vi "BOC_type-determain.vi"(0 "paramUnicorn_in":T4, 1 "UI_in":T1, 2 "TCP_conn":bool) -> (6 "paramUnicorn_out":T4={"conParam"={"ReadIntParam"=TRUE, "ReadDescrParam"=FALSE, "ReadFloatParam"=TRUE, "debug"=FALSE, "ReadJSON"=TRUE, "IP_address"="192.168.1.216", "N_attempts"=3, "type_con"=enum."TCP", "MB_address"=1, "VISA"="COM1", "connection ID"=refnum, "nameDevices"="", "timeout"=3000, "port"=2000, "type_version"="0F0C0001", "baud_rate"=115200, "VersionControl"=FALSE, "TCP_conn"=FALSE, "WindowSize"=700}, "Param"={"NumParam"={"NTelem"=0, "NInt"=0, "NFloat"=0, "NTable"=0}, "ParamInt"=[], "Telemetry"=[], "Table"=[], "ParamFloat"=[]}}, 7 "UI_out":T1)   [LabVIEW 2017]
uses:
  Unicorn Labview Library/Control/unicorn_Param.ctl
  Unicorn Labview Library/Control/unicorn_conn.ctl
  Unicorn Labview Library/Control/unicorn_JSON.ctl
  Unicorn Labview Library/Control/unicorn_ParamInt.ctl
  Unicorn Labview Library/Control/unicorn_Telemetry.ctl
  Unicorn Labview Library/Control/unicorn_Table.ctl
  Unicorn Labview Library/Control/unicorn_ParamFloat.ctl
  ui.ctl
  classes/dc_power_supply/DC_power_supply.lvclass
  classes/report/Report.lvclass
  ui_buttons.ctl
  types/boc_type.ctl
  <vilib>/regexp/Match Regular Expression.xnode
  Unicorn Labview Library/Unicorn Library.lvlib
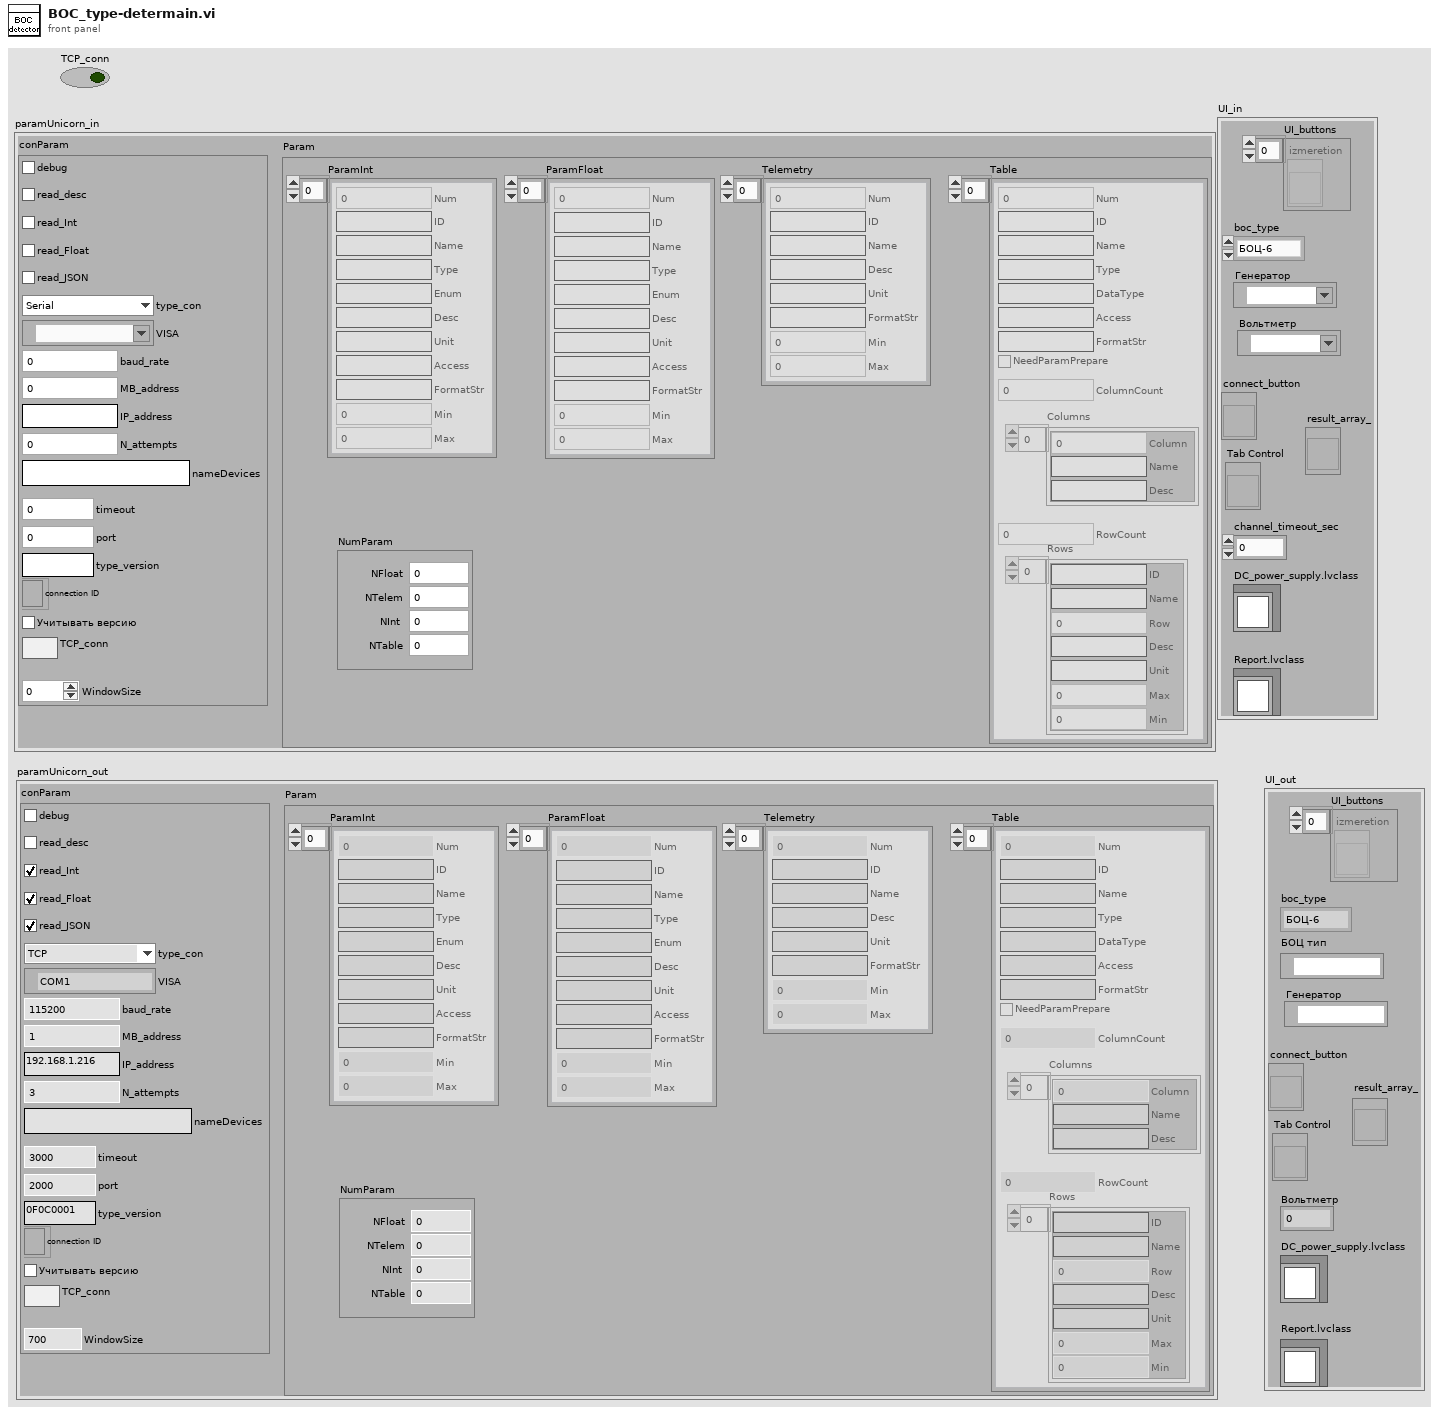
[diagram p1: front panel]
types:
  T1 = typedef "ui.ctl" = cluster{"UI_buttons":T2, "Tab Control":refnum<vi>, "connect_button":refnum<vi>, "generator":refnum<visa-resource-name>, "voltmetr":refnum<visa-resource-name>, "channel_timeout_sec":dbl, "boc_type":T3, "result_array_":refnum<vi>, "DC_power_supply.lvclass":refnum<class "DC_power_supply.lvclass">, "Report.lvclass":refnum<class "Report.lvclass">}
  T2 = typedef "ui_buttons.ctl" = refnum<vi>[]
  T3 = typedef "boc_type.ctl" = enum16{"БОЦ-6", "БОЦ-12"}
  T4 = typedef "Unicorn Library.lvlib/unicorn_Param.ctl" = cluster{"conParam":T5, "Param":T6}
  T5 = typedef "Unicorn Library.lvlib/unicorn_conn.ctl" = cluster{"ReadIntParam":bool, "ReadDescrParam":bool, "ReadFloatParam":bool, "debug":bool, "ReadJSON":bool, "IP_address":string, "N_attempts":i32, "type_con":enum16{"Serial", "TCP"}, "MB_address":i32, "VISA":refnum<visa-resource-name>, "connection ID":refnum<k5>, "nameDevices":string, "timeout":i32, "port":u16, "type_version":string, "baud_rate":u32, "VersionControl":bool, "TCP_conn":bool, "WindowSize":i32}
  T6 = typedef "Unicorn Library.lvlib/unicorn_JSON.ctl" = cluster{"NumParam":cluster{"NTelem":i32, "NInt":i32, "NFloat":i32, "NTable":i32}, "ParamInt":T7, "Telemetry":T8, "Table":T9, "ParamFloat":T10}
  T7 = typedef "Unicorn Library.lvlib/unicorn_ParamInt.ctl" = cluster{"ID":string, "Num":i32, "Name":string, "Type":string, "Enum":string, "Desc":string, "Unit":string, "Access":string, "FormatStr":string, "Min":i32, "Max":i32}[]
  T8 = typedef "Unicorn Library.lvlib/unicorn_Telemetry.ctl" = cluster{"ID":string, "Num":i32, "Name":string, "Desc":string, "Unit":string, "FormatStr":string, "Min":i32, "Max":i32}[]
  T9 = typedef "Unicorn Library.lvlib/unicorn_Table.ctl" = cluster{"Num":i32, "Access":string, "ColumnCount":i32, "NeedParamPrepare":bool, "Columns":cluster{"Column":i32, "Desc":string, "Name":string}[], "DataType":string, "FormatStr":string, "ID":string, "Name":string, "RowCount":i32, "Rows":cluster{"Desc":string, "ID":string, "Max":i32, "Min":i32, "Name":string, "Row":i32, "Unit":string}[], "Type":string}[]
  T10 = typedef "Unicorn Library.lvlib/unicorn_ParamFloat.ctl" = cluster{"ID":string, "Num":i32, "Name":string, "Type":string, "Enum":string, "Desc":string, "Unit":string, "Access":string, "FormatStr":string, "Min":i32, "Max":i32}[]
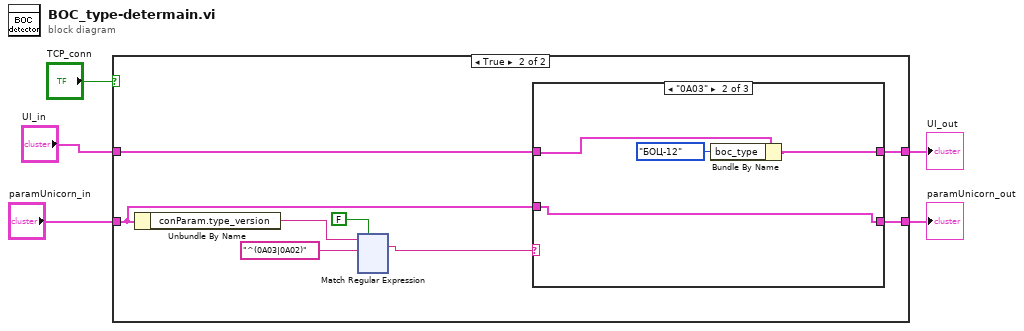
[diagram p0: block diagram]
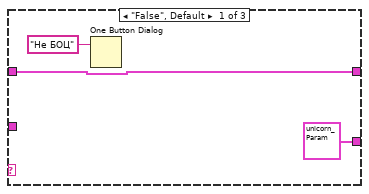
[diagram p3: hidden frame]
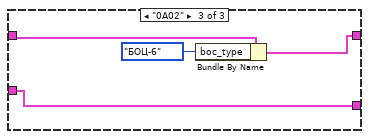
[diagram p4: hidden frame]
diagram:
  n1 = case shown="True" "TCP_conn" {
    tunnel: "paramUnicorn_in" -> [w7 w10]
    tunnel: "UI_in" -> [w6 w12]
    tunnel: [w6 w11] -> w3
    tunnel: [w7 w9] -> w2
    frame False {
    }
    frame True {
      n2 = Unbundle By Name(w10) -> ("conParam.type_version"=w15:string)
      n3 = xnode "Match Regular Expression"("input string"=w15, "regular expression"="^(0A03|0A02)", "ignore case? (F)"=FALSE) -> ("whole match"=w8:string)  [unwired: 3 in, 4 out]
      n4 = case shown="\"0A03\"" w8 {
        tunnel: w12 -> [w18 w21 w24]
        tunnel: [w18 w20 w23] -> w11
        tunnel: w10 -> [_ w19 w26]
        tunnel: [T4 {"conParam"={"ReadIntParam"=TRUE, "ReadDescrParam"=FALSE, "ReadFloatParam"=TRUE, "debug"=FALSE, "ReadJSON"=TRUE, "IP_address"="192.168.1.216", "N_attempts"=3, "type_con"=enum."TCP", "MB_address"=1, "VISA"="COM1", "connection ID"=refnum, "nameDevices"="", "timeout"=3000, "port"=2000, "type_version"="0F0C0001", "baud_rate"=115200, "VersionControl"=FALSE, "TCP_conn"=FALSE, "WindowSize"=700}, "Param"={"NumParam"={"NTelem"=0, "NInt"=0, "NFloat"=0, "NTable"=0}, "ParamInt"=[], "Telemetry"=[], "Table"=[], "ParamFloat"=[]}} ("paramUnicorn") w19 w26] -> w9
        frame "False", Default {
          n5 = One Button Dialog(message="Не БОЦ") -> ()  [unwired: 1 in, 1 out]
        }
        frame "0A03" {
          n6 = Bundle By Name(cluster=w21, "boc_type"=boc_type."БОЦ-12") -> (w20:T1)
        }
        frame "0A02" {
          n7 = Bundle By Name(cluster=w24, "boc_type"=boc_type."БОЦ-6") -> (w23:T1)
        }
      }
    }
  }
  "UI_out" <- w3
  "paramUnicorn_out" <- w2
